vi "Log AI.vi"(7 "AI\nAO\nDO\nTC\nACC\nStrain":refnum<queue>[](array[refnum]), 8 "error in":errorcluster, 11 "tdms file out":refnum<k34>) -> (0 "error out":errorcluster, 3 "tdms ref out":refnum<k34>)   [LabVIEW 2022 SP3]
uses:
  <vilib>/Waveform/WDTOps.llb/WDT Get Waveform Time Array DBL.vi
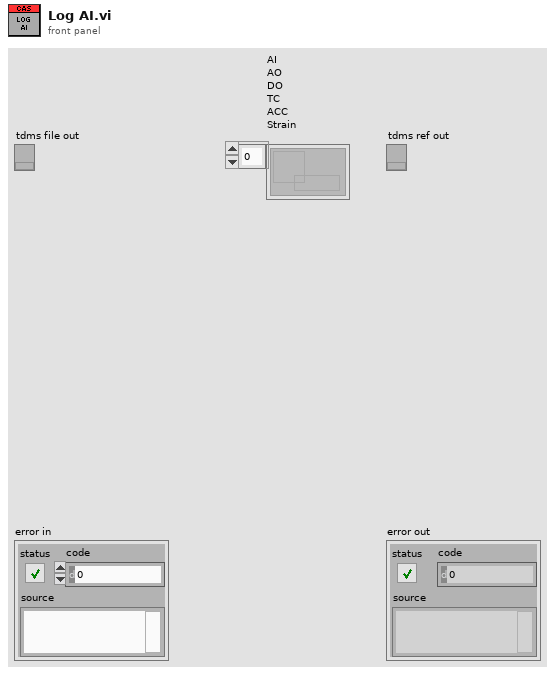
[diagram p1: front panel]
types:
  T1 = cluster{"AO Names":string[], "AI Names":string[], "DI Names":string[], "DO Names":string[], "TC Names":string[], "AO Default":dbl[], "DO Default":bool[], "ACC Names":string[], "SG Names":string[]}
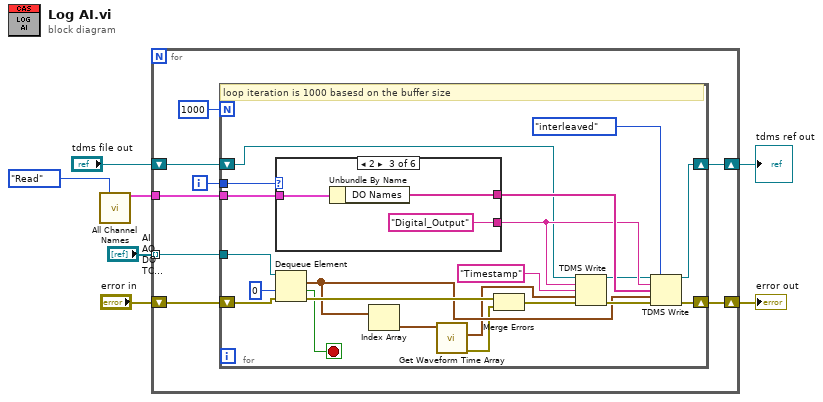
[diagram p0: block diagram]
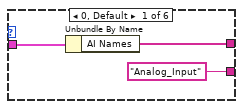
[diagram p2: hidden frame]
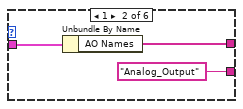
[diagram p3: hidden frame]
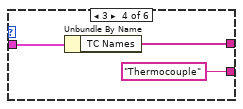
[diagram p4: hidden frame]
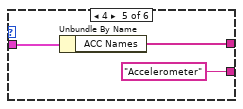
[diagram p5: hidden frame]
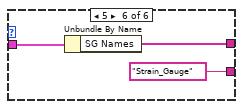
[diagram p6: hidden frame]
diagram:
  n1 = call "All Channel Names.vi"("Enum"=enum16{"Read", "Write"}."Read") -> ("Channel names"=w2:T1)  [unwired: 13 in, 1 out]
  n2 = for {
    tunnel: "AI\nAO\nDO\nTC\nACC\nStrain" -> [w14] mode=indexing
    shift-right: [w12] -> w5
    shift-left: "tdms file out" -> [w15]
    shift-right: [w10] -> w4
    shift-left: "error in" -> [w11]
    tunnel: w2 -> [w8]
    i -> [w9]
    n3 = for {
      N: 1000 -> [_]
      tunnel: w14 -> [w33]
      shift-right: [w25] -> w12
      shift-left: w15 -> [w27]
      shift-right: [w30] -> w10
      shift-left: w11 -> [w32]
      tunnel: w9 -> [w36]
      tunnel: w8 -> [w21]
      stop <- w23 stop-if-true
      # "loop iteration is 1000 basesd on the buffer size"
      n4 = case shown="2" w36 {
        tunnel: [w38 w40 w43 w46 w49 w52] -> w29
        tunnel: ["Analog_Input" ("group name in (Untitled)") "Analog_Output" ("group name in (Untitled)") "Digital_Output" ("group name in (Untitled)") "Thermocouple" ("group name in (Untitled)") "Accelerometer" ("group name in (Untitled)") "Strain_Gauge" ("group name in (Untitled)")] -> w28
        tunnel: w21 -> [w37 w41 w44 w47 w50 w53]
        frame 0, Default {
          n5 = Unbundle By Name(w37) -> ("AI Names"=w38:string[])
        }
        frame 1 {
          n6 = Unbundle By Name(w41) -> ("AO Names"=w40:string[])
        }
        frame 2 {
          n7 = Unbundle By Name(w44) -> ("DO Names"=w43:string[])
        }
        frame 3 {
          n8 = Unbundle By Name(w47) -> ("TC Names"=w46:string[])
        }
        frame 4 {
          n9 = Unbundle By Name(w50) -> ("ACC Names"=w49:string[])
        }
        frame 5 {
          n10 = Unbundle By Name(w53) -> ("SG Names"=w52:string[])
        }
      }
      n11 = Dequeue Element(queue=w33, timeout in ms (-1)=0, error in (no error)=w32) -> (element=w24:waveform(dbl)[], timed out?=w23:bool, error out=w34:errorcluster)  [unwired: 1 out]
      n12 = Index Array(array=w24) -> (element=w19:waveform(dbl))  [unwired: 1 in]
      n13 = call-poly <vilib>:"Get Waveform Time Array.vi"("waveform in"=w19) -> ("error out"=w20:errorcluster, "X array"=w16:timestamp[])  [unwired: 9 in]
      n14 = Merge Errors(w34, w20) -> (w18:errorcluster)
      n15 = TDMS Write(0:w27, 5:w28, 7:"Timestamp", 9:w16, 11:w18) -> (4:w26:refnum<k34>, 15:w31:errorcluster)  [unwired: 1 in, 2 out]
      n16 = TDMS Write(0:w26, 1:enum16{"decimated", "interleaved"}."interleaved" ("data layout (0:decimated)"), 5:w28, 7:w29, 9:w24, 11:w31) -> (4:w25:refnum<k34>, 15:w30:errorcluster)  [unwired: 2 out]
    }
  }
  "tdms ref out" <- w5
  "error out" <- w4
